vi "e.gate Tree.vi"   [LabVIEW 2016]
doc: "<B>AMC - Analytik & Messtechnik GmbH Chemnitz</B>\n\nLabVIEW Drivers for e.gate/e.pac series from Gantner Instruments\n\nThe VI Tree displays all the user-callable VIs of the instrument driver in an organized table. It isn't executable and only for overview."
uses:
  e.gate ASCII Write Value - Boolean.vi
  e.gate HighSpeedPort Get File - Read Directory.vi
  e.gate ASCII Read Value - Double.vi
  e.gate HighSpeedPort Diagnostics Full.vi
  e.gate Decode UDBF - File.vi
panel:
  # "SEE DIAGRAM\nFOR VI TREE."
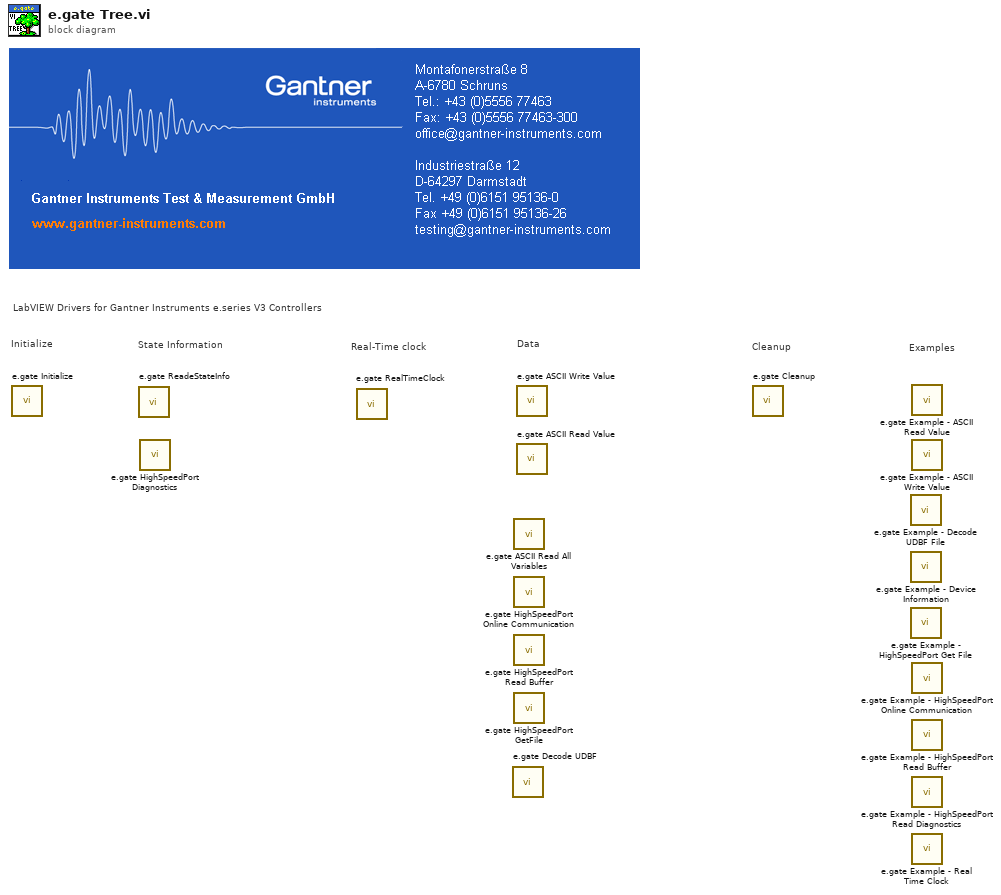
[diagram p0: block diagram]
diagram:
  # "Examples"
  # "Real-Time clock"
  # "LabVIEW Drivers for Gantner Instruments e.series V3 Controllers"
  # "Data"
  # "State Information"
  # "Cleanup"
  # "Initialize"
  n1 = call "e.gate Initialize.vi"() -> ()  [unwired: 10 in, 2 out]
  n2 = call "e.gate ReadeStateInfo.vi"() -> ()  [unwired: 14 in, 6 out]
  n3 = call-poly "e.gate HighSpeedPort Diagnostics.vi"() -> ()  [unwired: 11 in, 5 out]
  n4 = call "e.gate RealTimeClock.vi"() -> ()  [unwired: 25 in, 3 out]
  n5 = call-poly "e.gate Decode UDBF.vi"() -> ()  [unwired: 9 in, 3 out]
  n6 = call "e.gate ASCII Read All Variables.vi"() -> ()  [unwired: 9 in, 3 out]
  n7 = call "e.gate HighSpeedPort Online Communication.vi"() -> ()  [unwired: 9 in, 3 out]
  n8 = call "e.gate HighSpeedPort Read Buffer.vi"() -> ()  [unwired: 13 in, 3 out]
  n9 = call-poly "e.gate HighSpeedPort GetFile.vi"() -> ()  [unwired: 9 in, 3 out]
  n10 = call-poly "e.gate ASCII Write Value.vi"() -> ()  [unwired: 10 in, 2 out]
  n11 = call-poly "e.gate ASCII Read Value.vi"() -> ()  [unwired: 9 in, 3 out]
  n12 = call "e.gate Cleanup.vi"() -> ()  [unwired: 11 in, 1 out]
  n13 = call "e.gate Example - Decode UDBF File.vi"() -> ()  [unwired: 1 in]
  n14 = call "e.gate Example - Device Information.vi"() -> ()  [unwired: 1 in]
  n15 = call "e.gate Example - HighSpeedPort Get File.vi"() -> ()  [unwired: 1 in]
  n16 = call "e.gate Example - ASCII Read Value.vi"() -> ()  [unwired: 11 in, 1 out]
  n17 = call "e.gate Example - ASCII Write Value.vi"() -> ()  [unwired: 1 in]
  n18 = call "e.gate Example - HighSpeedPort Online Communication.vi"() -> ()  [unwired: 11 in, 1 out]
  n19 = call "e.gate Example - HighSpeedPort Read Buffer.vi"() -> ()  [unwired: 11 in, 1 out]
  n20 = call "e.gate Example - HighSpeedPort Read Diagnostics.vi"() -> ()  [unwired: 1 in]
  n21 = call "e.gate Example - Real Time Clock.vi"() -> ()  [unwired: 1 in]
